vi "GetStatus.vi"(8 "error in (no error)":errorcluster, 11 "GS in":refnum<class "GuiderSetup.lvclass">) -> (0 "error out":errorcluster, 3 "GS out":refnum<class "GuiderSetup.lvclass">)   [LabVIEW 2018, in "GuiderSetup.lvclass"]
uses:
  GuiderSetup.lvclass
  C:/Users/devstaff/sparc4/s4gui/Versao ZeroMQ REQ-REP/SPARC4_GUI -v1.0.8 - reconhecimento do ACK do ACS/S4GUI/S4GUI.lvclass
  S4GUI/S4GUI.lvclass/S4GUI.ctl
  Instrument/Instrument.lvclass/Instrument.ctl
  Device/Optics/Optics.lvclass/Optics.ctl
  Server/Server.lvclass/Server.ctl
  Device/Optics/Opt_Continuous/Opt_Continuous.lvclass
  C:/Users/devstaff/sparc4/s4gui/Versao ZeroMQ REQ-REP/SPARC4_GUI -v1.0.8 - reconhecimento do ACK do ACS/Device/Optics/Optics.lvclass
  Instrument/Instrument.lvclass
  C:/Users/devstaff/sparc4/s4gui/Versao ZeroMQ REQ-REP/SPARC4_GUI -v1.0.8 - reconhecimento do ACK do ACS/Server/Server.lvclass
  S4GUI/S4GUI.lvclass
  Device/Optics/Optics.lvclass
  Server/Server.lvclass
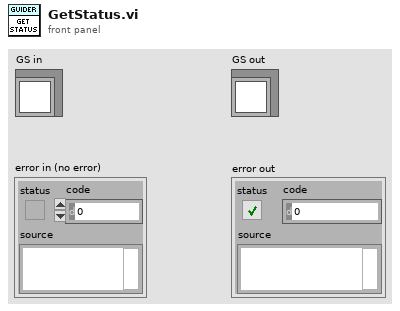
[diagram p1: front panel]
types:
  T1 = cluster{"Trigger Mode Status":string, "String output":string, "Instrument Status":cluster{"WPROT pos":dbl, "WPSEL pos":dbl, "GMIR pos":dbl, "GFOC pos":dbl, "CALW pos":dbl, "ASEL pos":dbl, "mode":bool, "String Status":string, "connection":bool, "operational":bool}, "Sync Box State":i32, "Trigger General Status":string, "Instrument States":cluster{"WPSEL State":i32, "WPROT State":i32, "CALW State":i32, "ASEL State":i32, "GMIR State":i32, "GFOC State":i32}, "Instrument Pos Names":cluster{"WPROT posname":string, "WPSEL posname":string, "CALW posname":string, "ASEL posname":string}, "ChannelA_Status":cluster{"Current exp":dbl, "Frames done":u32, "LastFileImage":string, "CamStatus":string, "Run state":u32, "connection":bool, "Cooler ON/OFF":i16, "Currently temperature":i16, "Temperature Status":string, "target  temp":i16, "conf runing":bool, "FT":bool, "UsedDisk":u16, "operational":bool}, "WPROT seq":u16, "ChannelB_Status":cluster{"Current exp":dbl, "Frames done":u32, "LastFileImage":string, "CamStatus":string, "Run state":u32, "connection":bool, "Cooler ON/OFF":i16, "Currently temperature":i16, "Temperature Status":string, "target  temp":i16, "conf runing":bool, "FT":bool, "UsedDisk":u16, "operational":bool}, "ChannelC_Status":cluster{"Current exp":dbl, "Frames done":u32, "LastFileImage":string, "CamStatus":string, "Run state":u32, "connection":bool, "Cooler ON/OFF":i16, "Currently temperature":i16, "Temperature Status":string, "target  temp":i16, "conf runing":bool, "FT":bool, "UsedDisk":u16, "operational":bool}, "ChannelD_Status":cluster{"Current exp":dbl, "Frames done":u32, "LastFileImage":string, "CamStatus":string, "Run state":u32, "connection":bool, "Cooler ON/OFF":i16, "Currently temperature":i16, "Temperature Status":string, "target  temp":i16, "conf runing":bool, "FT":bool, "UsedDisk":u16, "operational":bool}, "ChannelA_CCD":cluster{"ACQUISITION_MODE":u8, "TRIGGER_MODE":u8, "READ_MODE":u8, "PREAMP":u8, "READOUT_RATE":u8, "VERTICAL_SHIFT_SPEED":u8, "EM_MODE":u8, "EM_GAIN":u16, "SHUTTER_MODE":u8, "SHUTTER_TTL":u8, "SHUTTER_OPENNING_TIME":u16, "SHUTTER_CLOSING_TIME":u16, "VBIN":u16, "HBIN":u16, "INITIAL_LINE":u16, "INITIAL_COLUMN":u16, "FINAL_LINE":u16, "FINAL_COLUMN":u16, "FRAME_TRANSFER":bool, "VERTICAL_CLOCK_VOLTAGE":u8, "AD_CHANNEL":u32}, "ChannelB_CCD ":cluster{"ACQUISITION_MODE":u8, "TRIGGER_MODE":u8, "READ_MODE":u8, "PREAMP":u8, "READOUT_RATE":u8, "VERTICAL_SHIFT_SPEED":u8, "EM_MODE":u8, "EM_GAIN":u16, "SHUTTER_MODE":u8, "SHUTTER_TTL":u8, "SHUTTER_OPENNING_TIME":u16, "SHUTTER_CLOSING_TIME":u16, "VBIN":u16, "HBIN":u16, "INITIAL_LINE":u16, "INITIAL_COLUMN":u16, "FINAL_LINE":u16, "FINAL_COLUMN":u16, "FRAME_TRANSFER":bool, "VERTICAL_CLOCK_VOLTAGE":u8, "AD_CHANNEL":u32}, "ChannelC_CCD":cluster{"ACQUISITION_MODE":u8, "TRIGGER_MODE":u8, "READ_MODE":u8, "PREAMP":u8, "READOUT_RATE":u8, "VERTICAL_SHIFT_SPEED":u8, "EM_MODE":u8, "EM_GAIN":u16, "SHUTTER_MODE":u8, "SHUTTER_TTL":u8, "SHUTTER_OPENNING_TIME":u16, "SHUTTER_CLOSING_TIME":u16, "VBIN":u16, "HBIN":u16, "INITIAL_LINE":u16, "INITIAL_COLUMN":u16, "FINAL_LINE":u16, "FINAL_COLUMN":u16, "FRAME_TRANSFER":bool, "VERTICAL_CLOCK_VOLTAGE":u8, "AD_CHANNEL":u32}, "ChannelD_CCD":cluster{"ACQUISITION_MODE":u8, "TRIGGER_MODE":u8, "READ_MODE":u8, "PREAMP":u8, "READOUT_RATE":u8, "VERTICAL_SHIFT_SPEED":u8, "EM_MODE":u8, "EM_GAIN":u16, "SHUTTER_MODE":u8, "SHUTTER_TTL":u8, "SHUTTER_OPENNING_TIME":u16, "SHUTTER_CLOSING_TIME":u16, "VBIN":u16, "HBIN":u16, "INITIAL_LINE":u16, "INITIAL_COLUMN":u16, "FINAL_LINE":u16, "FINAL_COLUMN":u16, "FRAME_TRANSFER":bool, "VERTICAL_CLOCK_VOLTAGE":u8, "AD_CHANNEL":u32}, "CHA_Checked Params":cluster{"ACQUISITION_MODE":bool, "TRIGGER_MODE":bool, "READ_MODE":bool, "PREAMP":bool, "READOUT_RATE":bool, "VERTICAL_SHIFT_SPEED":bool, "EM_MODE":bool, "EM_GAIN":bool, "SHUTTER_MODE":bool, "SHUTTER_TTL":bool, "SHUTTER_OPENING_TIME":bool, "SHUTTER_CLOSING_TIME":bool, "VBIN":bool, "HBIN":bool, "INITIAL_LINE":bool, "INITIAL_COLUMN":bool, "FINAL_LINE":bool, "FINAL_COLUMN":bool, "FRAME_TRANSFER":bool, "VERTICAL_CLOCK_VOLTAGE":bool, "AD_CHANNEL":bool}, "CHB_Checked Params":cluster{"ACQUISITION_MODE":bool, "TRIGGER_MODE":bool, "READ_MODE":bool, "PREAMP":bool, "READOUT_RATE":bool, "VERTICAL_SHIFT_SPEED":bool, "EM_MODE":bool, "EM_GAIN":bool, "SHUTTER_MODE":bool, "SHUTTER_TTL":bool, "SHUTTER_OPENING_TIME":bool, "SHUTTER_CLOSING_TIME":bool, "VBIN":bool, "HBIN":bool, "INITIAL_LINE":bool, "INITIAL_COLUMN":bool, "FINAL_LINE":bool, "FINAL_COLUMN":bool, "FRAME_TRANSFER":bool, "VERTICAL_CLOCK_VOLTAGE":bool, "AD_CHANNEL":bool}, "CHC_Checked Params":cluster{"ACQUISITION_MODE":bool, "TRIGGER_MODE":bool, "READ_MODE":bool, "PREAMP":bool, "READOUT_RATE":bool, "VERTICAL_SHIFT_SPEED":bool, "EM_MODE":bool, "EM_GAIN":bool, "SHUTTER_MODE":bool, "SHUTTER_TTL":bool, "SHUTTER_OPENING_TIME":bool, "SHUTTER_CLOSING_TIME":bool, "VBIN":bool, "HBIN":bool, "INITIAL_LINE":bool, "INITIAL_COLUMN":bool, "FINAL_LINE":bool, "FINAL_COLUMN":bool, "FRAME_TRANSFER":bool, "VERTICAL_CLOCK_VOLTAGE":bool, "AD_CHANNEL":bool}, "CHD_Checked Params":cluster{"ACQUISITION_MODE":bool, "TRIGGER_MODE":bool, "READ_MODE":bool, "PREAMP":bool, "READOUT_RATE":bool, "VERTICAL_SHIFT_SPEED":bool, "EM_MODE":bool, "EM_GAIN":bool, "SHUTTER_MODE":bool, "SHUTTER_TTL":bool, "SHUTTER_OPENING_TIME":bool, "SHUTTER_CLOSING_TIME":bool, "VBIN":bool, "HBIN":bool, "INITIAL_LINE":bool, "INITIAL_COLUMN":bool, "FINAL_LINE":bool, "FINAL_COLUMN":bool, "FRAME_TRANSFER":bool, "VERTICAL_CLOCK_VOLTAGE":bool, "AD_CHANNEL":bool}, "Trigger_connection":bool, "TCSPD_connection":bool, "TCS extended":string, "TCS id":u32, "S4ICS id":u32, "focus pos":i32, "Focus_connection":bool, "WS_connection":bool, "weather status":cluster{"broker":string, "version":string, "date":string, "hour":string, "outHumidity":string, "inHumidity":string, "inTemp":string, "outTemp":string, "windSpeed":string, "windDirection":string, "pressure":string, "dewOut":string, "dewIn":string, "leaf":string, "rain":string, "windChill":string}, "GS STATUS cluster":cluster{"FocusPhot":dbl, "FocusPolar":dbl, "FocusEffic":dbl, "FocusInstrum":dbl, "ICS":bool, "AG":bool, "BROKER":string, "timestamp":string, "FocusPos":dbl, "MirrorPos":dbl}, "TCSPD_operational":bool, "Focus_operational":bool, "object_suffix":string, "dflat_suffix":string, "sflat_suffix":string, "dark_suffix":string, "zero_suffix":string, "focus_suffix":string, "suffixAlertVisible":bool, "Instrument Motor error":cluster{"WPSEL error":bool, "WPROT error":bool, "CALW error":bool, "ASEL error":bool, "GMIR error":bool, "GFOC error":bool}}
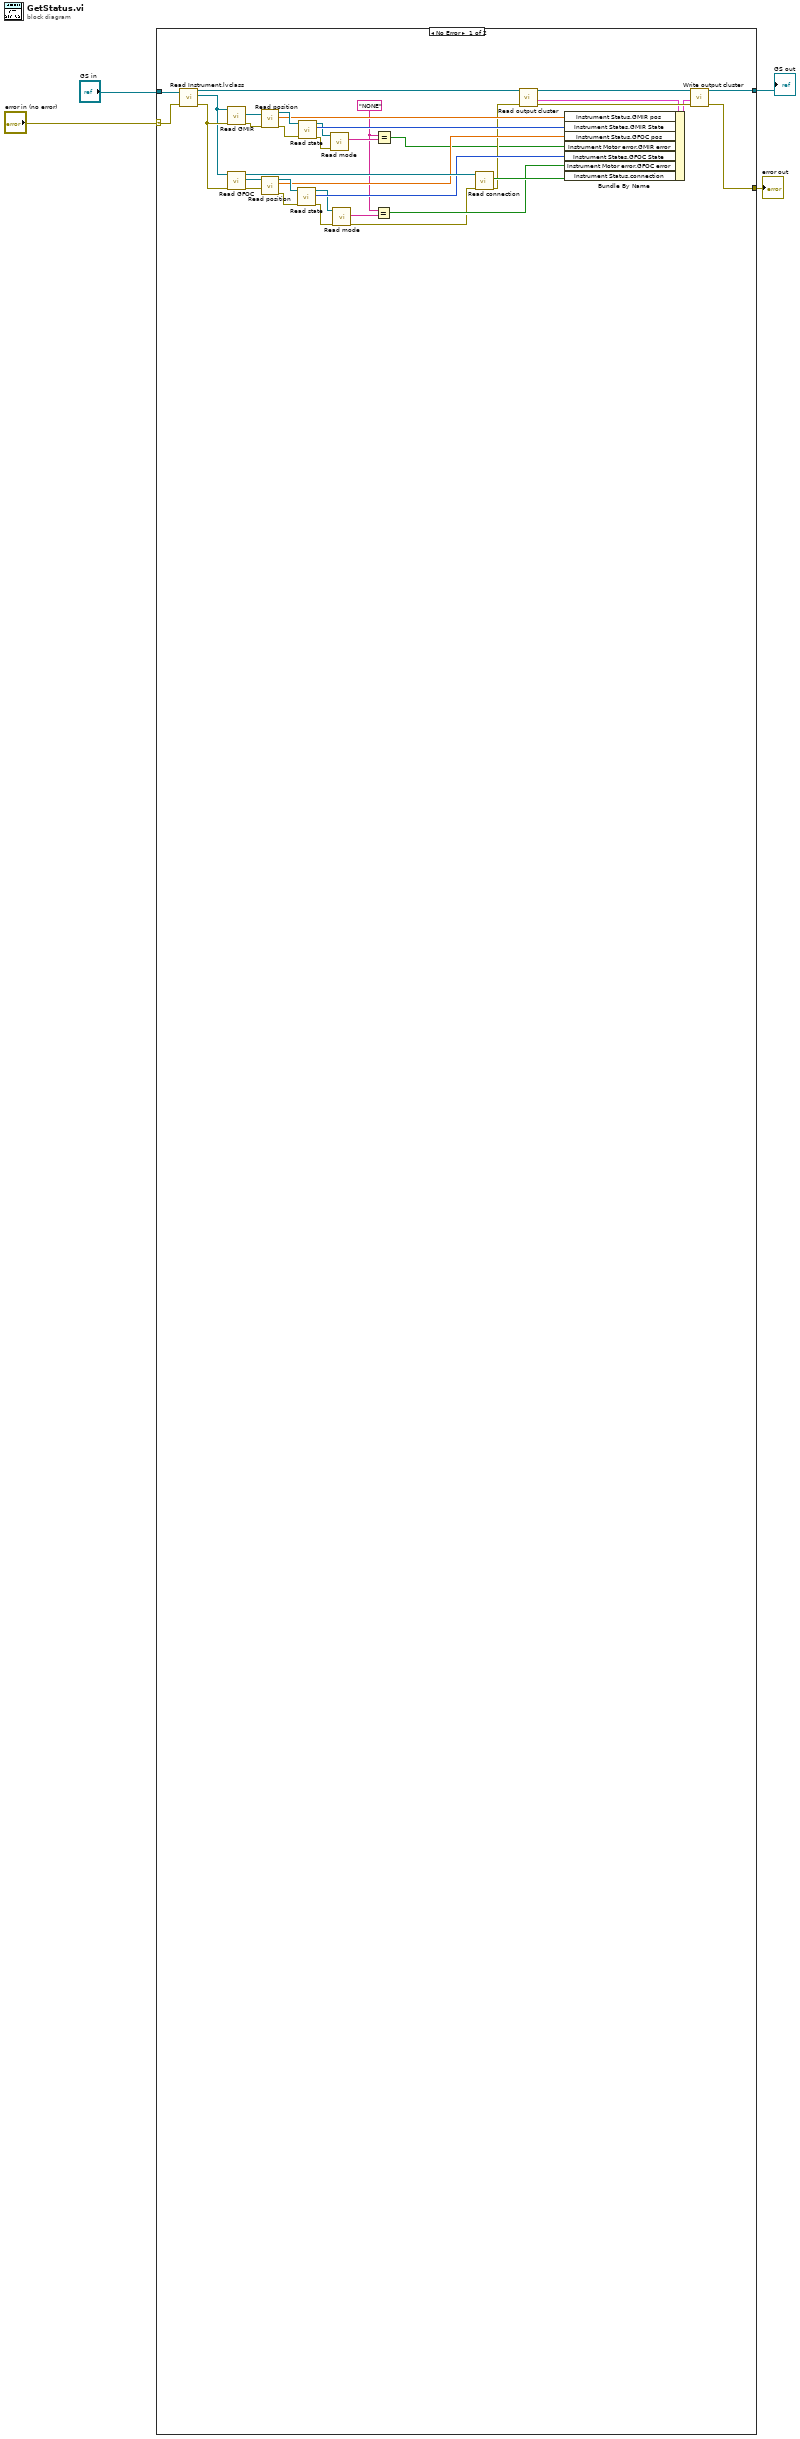
[diagram p0: block diagram]
diagram:
  n1 = case shown="No Error" "error in (no error)" {
    selector: "error in (no error)" -> [w30 w41]
    tunnel: "GS in" -> [w29 w42]
    tunnel: [w22 w42] -> w2
    tunnel: [w21 w41] -> w1
    frame No Error {
      w7 = "NONE"
      n2 = call "Read Instrument.lvclass.vi"("error in (no error)"=w30, "S4ACS_GUI in"=w29) -> ("error out"=w31:errorcluster, "Instrument.lvclass"=w28:refnum<class "Instrument.lvclass">, "S4ACS_GUI out"=w20:refnum<class "GuiderSetup.lvclass">)  [unwired: 7 in]
      n3 = call "Read GMIR.vi"("error in (no error)"=w31, "Instrument in"=w28) -> ("error out"=w40:errorcluster, "Opt_Continuous.lvclass"=w39:refnum<class "Opt_Continuous.lvclass">)  [unwired: 7 in, 1 out]
      n4 = call "Read GFOC.vi"("error in (no error)"=w31, "Instrument in"=w28) -> ("error out"=w37:errorcluster, "Opt_Continuous.lvclass"=w38:refnum<class "Opt_Continuous.lvclass">, "Instrument out"=w32:refnum<class "Instrument.lvclass">)  [unwired: 7 in]
      n5 = call "Read position.vi"("error in (no error)"=w40, "Optics in"=w39) -> ("error out"=w35:errorcluster, "position"=w26:dbl, "Optics out"=w36:refnum<class "Opt_Continuous.lvclass">)  [unwired: 7 in]
      n6 = call "Read position.vi"("error in (no error)"=w37, "Optics in"=w38) -> ("error out"=w33:errorcluster, "position"=w24:dbl, "Optics out"=w34:refnum<class "Opt_Continuous.lvclass">)  [unwired: 7 in]
      n7 = call-dynamic "Read state.vi"("error in (no error)"=w33, "Optics in"=w34) -> ("error out"=w9:errorcluster, "state"=w23:u8, "Optics out"=w8:refnum<class "Opt_Continuous.lvclass">)  [unwired: 7 in]
      n8 = call-dynamic "Read state.vi"("error in (no error)"=w35, "Optics in"=w36) -> ("error out"=w13:errorcluster, "state"=w25:u8, "Optics out"=w14:refnum<class "Opt_Continuous.lvclass">)  [unwired: 7 in]
      n9 = call "Read mode.vi"("error in (no error)"=w13, "Optics in"=w14) -> ("mode"=w12:string)  [unwired: 7 in, 2 out]
      n10 = call "Read mode.vi"("error in (no error)"=w9, "Optics in"=w8) -> ("error out"=w5:errorcluster, "mode"=w10:string)  [unwired: 7 in, 1 out]
      n11 = Equal?(x=w7, y=w10) -> (x = y?=w6:bool)
      n12 = Equal?(x=w7, y=w12) -> (x = y?=w11:bool)
      n13 = call "Read connection.vi"("error in (no error)"=w5, "Server in"=w32) -> ("error out"=w18:errorcluster, "connection"=w27:bool)  [unwired: 7 in, 1 out]
      n14 = call-dynamic "Read output cluster.vi"("error in (no error)"=w18, "S4GUI in"=w20) -> ("error out"=w17:errorcluster, "output cluster"=w16:T1, "S4GUI out"=w19:refnum<class "GuiderSetup.lvclass">)  [unwired: 7 in]
      n15 = Bundle By Name(cluster=w16, "Instrument Status.GMIR pos"=w26, "Instrument States.GMIR State"=w25, "Instrument Status.GFOC pos"=w24, "Instrument Motor error.GMIR error"=w11, "Instrument States.GFOC State"=w23, "Instrument Motor error.GFOC error"=w6, "Instrument Status.connection"=w27) -> (w15:T1)
      n16 = call-dynamic "Write output cluster.vi"("error in (no error)"=w17, "output cluster"=w15, "S4GUI in"=w19) -> ("error out"=w21:errorcluster, "S4GUI out"=w22:refnum<class "GuiderSetup.lvclass">)  [unwired: 7 in]
    }
    frame Error {
    }
  }
  "GS out" <- w2
  "error out" <- w1
